vi "Set Cursor Unbusy.vi"(8 "error in (no error)":errorcluster, 11 "IViewable In":refnum<class "IViewable.lvclass">) -> (0 "error out":errorcluster, 3 "IViewable Out":refnum<class "IViewable.lvclass">)   [LabVIEW 2020, in "IViewable.lvlib" / "IViewable.lvclass"]
doc: "设置光标取消忙碌"
uses:
  IViewable.lvclass
  IViewable.lvclass/IViewable.ctl
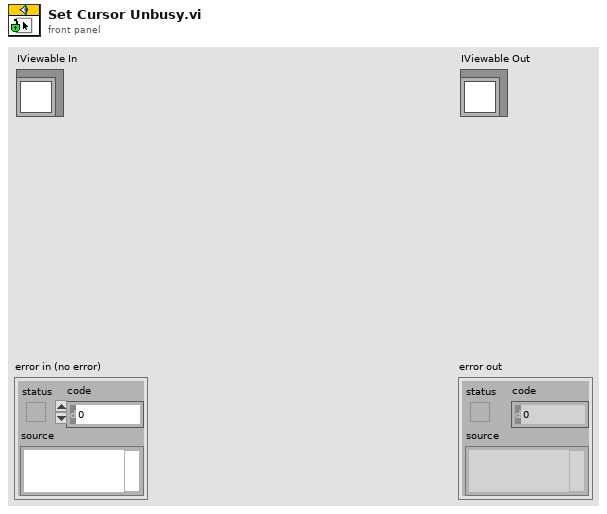
[diagram p1: front panel]
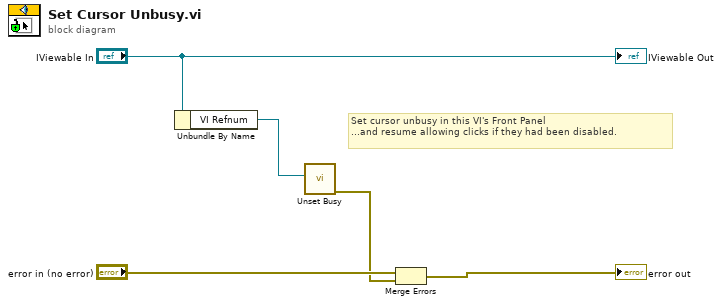
[diagram p0: block diagram]
diagram:
  # "Set cursor unbusy in this VI's Front Panel\n...and resume allowing clicks if they had been disabled."
  n1 = Unbundle By Name("IViewable In") -> ("VI Refnum"=w2:refnum<vi>)
  n2 = call <vilib>:"Unset Busy.vi"("VI reference (current VI)"=w2) -> ("error out"=w1:errorcluster)  [unwired: 10 in]
  n3 = Merge Errors("error in (no error)", w1) -> (→"error out":errorcluster)
  "IViewable Out" <- "IViewable In"
